vi "Cron Days.vi"(7 "Cron":refnum<class "Cron.lvclass">, 10 "Cron":T1) -> (2 "Cron Time":T1)   [LabVIEW 2013, in "openCron.lvlib" / "Cron.lvclass"]
uses:
  Cron.lvclass
  CronTime -- cluster.ctl
  Cron Interval -- enum.ctl
  Cron.lvclass/Cron.ctl
  <vilib>/LabVIEW Open Source Project/Epoch Date & Time/GregorianCal_Month -- enum.ctl
  <vilib>/LabVIEW Open Source Project/Epoch Date & Time/GregorianCal_MonthLengths.vi
  <vilib>/LabVIEW Open Source Project/Epoch Date & Time/isLeapYear (integer).vi
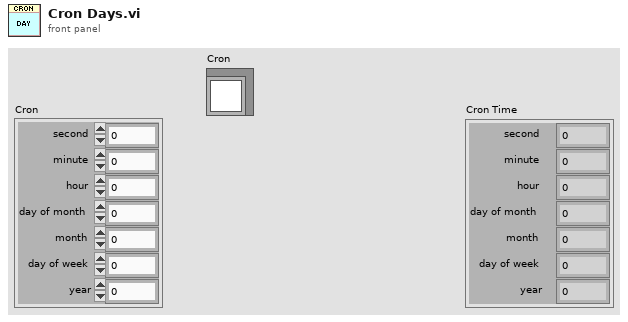
[diagram p1: front panel]
types:
  T1 = typedef "openCron.lvlib/Cron.lvclass/CronTime -- cluster.ctl" = cluster{"second":i32, "minute":i32, "hour":i32, "day of month":i32, "month":i32, "day of week":i32, "year":i32}
  T2 = typedef "openCron.lvlib/Cron.lvclass/Cron Interval -- enum.ctl" = enum16{"Seconds", "Minutes", "Hours", "Day of Month", "Month", "Day of Week", "Year"}
  T3 = typedef "openCron.lvlib/Cron.lvclass/Cron Interval -- cluster.ctl" = cluster{"Values":i32[], "All":bool, "Any":bool}
  T4 = typedef "GregorianCal_Month -- enum.ctl" = enum16{"January", "February", "March", "April", "May", "June", "July", "August", "September", "October", "November", "December"}
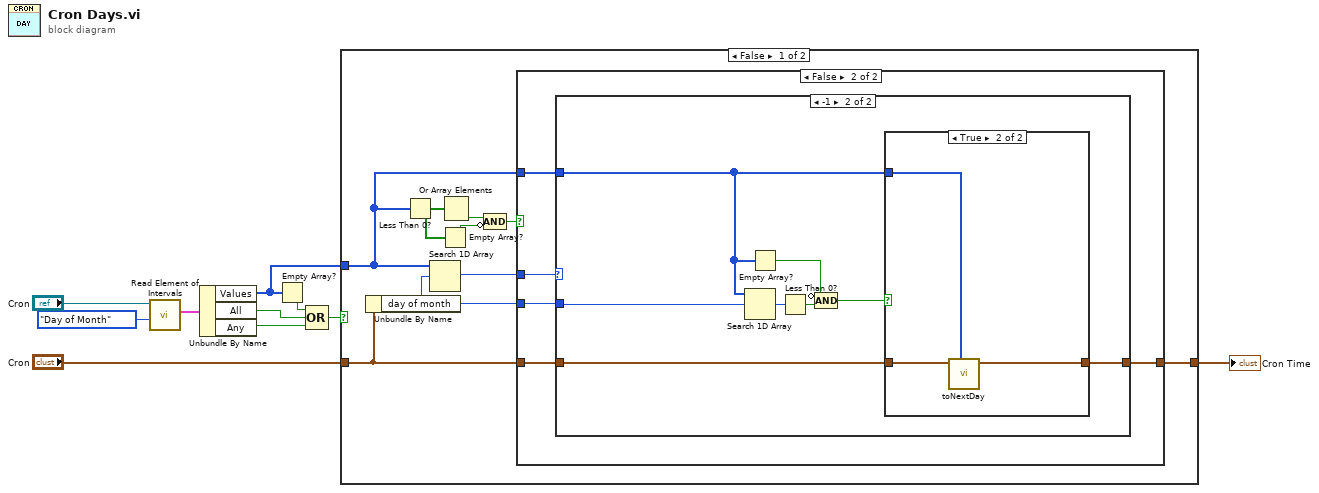
[diagram p0: block diagram]
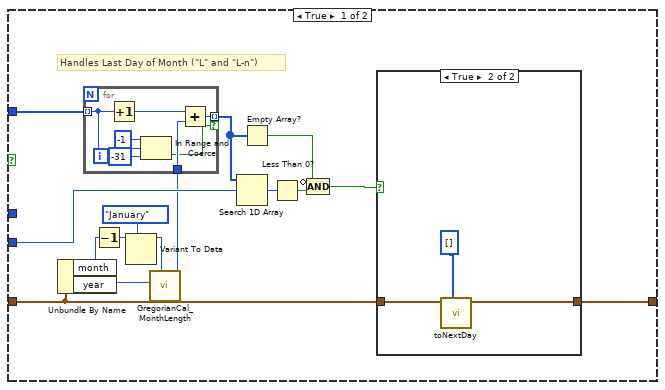
[diagram p2: hidden frame]
diagram:
  n1 = call "Read Element of Intervals.vi"("Interval"=Cron_Interval_--_enum."Day of Month", "Cron in"="Cron") -> ("Interval"=w6:T3)  [unwired: 7 in, 2 out]
  n2 = Unbundle By Name(w6) -> ("Values"=w1:i32[], "All"=w4:bool, "Any"=w5:bool)
  n3 = Empty Array?(array=w1) -> (empty?=w3:bool)
  n4 = Compound Arithmetic op=OR(w3, w4, w5) -> (w2:bool)
  n5 = case shown="False" w2 {
    tunnel: [w18 w64] -> w8
    tunnel: "Cron" -> [w19 w64]
    tunnel: w1 -> [w15 _]
    frame False {
      n6 = Unbundle By Name(w19) -> ("day of month"=w17:i32)
      n7 = Less Than 0?(x=w15) -> (x < 0?=w14:bool[])
      n8 = Search 1D Array(1D array=w15, element=w17) -> (index of element=w16:i32)  [unwired: 1 in]
      n9 = Empty Array?(array=w14) -> (empty?=w12:bool)
      n10 = Or Array Elements(Boolean array=w14) -> (logical OR=w13:bool)
      n11 = Compound Arithmetic op=AND(w13, invert w12) -> (w11:bool)
      n12 = case shown="False" w11 {
        tunnel: w19 -> [w34 w50]
        tunnel: [w33 w49] -> w18
        tunnel: w17 -> [w32 w48]
        tunnel: w16 -> [_ w47]
        tunnel: w15 -> [w31 w46]
        frame True {
          # "Handles Last Day of Month (\"L\" and \"L-n\")"
          n13 = Unbundle By Name(w34) -> ("month"=w29:i32, "year"=w30:i32)
          n14 = Decrement(x=w29) -> (x-1=w26:i32)
          n15 = Variant To Data(type=GregorianCal_Month_--_enum."January" ("Month"), Variant=w26) -> (data=w27:T4)  [unwired: 1 in, 1 out]
          n16 = call <vilib>:"GregorianCal_MonthLength.vi"("Month"=w27, "Year (0: this year)"=w30) -> ("Nb Days"=w25:i32)  [unwired: 9 in]
          n17 = for {
            tunnel: w31 -> [w38] mode=indexing
            tunnel: w25 -> [w40]
            tunnel: [w39] -> w23 mode=indexing if=w36
            n18 = Increment(x=w38) -> (x+1=w41:i32)
            n19 = In Range and Coerce(upper limit=-1, x=w38, lower limit=-31) -> (In Range?=w36:bool)  [unwired: 1 out]
            n20 = Add(x=w41, y=w40) -> (x+y=w39:i32)
          }
          n21 = Search 1D Array(1D array=w23, element=w32) -> (index of element=w24:i32)  [unwired: 1 in]
          n22 = Empty Array?(array=w23) -> (empty?=w22:bool)
          n23 = Less Than 0?(x=w24) -> (x < 0?=w21:bool)
          n24 = Compound Arithmetic op=AND(invert w22, w21) -> (w20:bool)
          n25 = case shown="True" w20 {
            tunnel: w34 -> [w42 w45]
            tunnel: [w42 w44] -> w33
            frame False {
            }
            frame True {
              n26 = call "toNextDay.vi"("Values"=i32[] [], "Cron in"=w45) -> ("Cron out"=w44:T1)  [unwired: 9 in]
            }
          }
        }
        frame False {
          n27 = case shown="-1" w47 {
            tunnel: w50 -> [w51 w58]
            tunnel: [w51 w59] -> w49
            tunnel: w48 -> [_ w57]
            tunnel: w46 -> [_ w52]
            frame Default {
            }
            frame -1 {
              n28 = Search 1D Array(1D array=w52, element=w57) -> (index of element=w56:i32)  [unwired: 1 in]
              n29 = Empty Array?(array=w52) -> (empty?=w55:bool)
              n30 = Less Than 0?(x=w56) -> (x < 0?=w54:bool)
              n31 = Compound Arithmetic op=AND(invert w55, w54) -> (w53:bool)
              n32 = case shown="True" w53 {
                tunnel: w58 -> [w60 w63]
                tunnel: [w60 w62] -> w59
                tunnel: w52 -> [_ w61]
                frame False {
                }
                frame True {
                  n33 = call "toNextDay.vi"("Values"=w61, "Cron in"=w63) -> ("Cron out"=w62:T1)  [unwired: 9 in]
                }
              }
            }
          }
        }
      }
    }
    frame True {
    }
  }
  "Cron Time" <- w8
